vi "DOCK_save_database_password.vi"(7 "error_in":errorcluster, 9 "new_password":string, 10 "all_config_info_in":T1={"main_ini_file"={"SQL Driver"="", "SQL Server"="", "SQL Database"="", "SQL UID"="", "Reference table"="", "Reference history"="", "Archivisation CFG table"="", "Archivisation CFG history"="", "User table"="", "User history"="", "default language"="", "SCANNER COM port"=0, "SCANNER Baud rate"=0, "SCANNER Data bits"=0, "SCANNER Pairity"=enum."None", "SCANNER Stop bits"=0, "SCANNER Flow control"=0, "SCANNER Termination char"=10, "PRINTER PC port"=0, "PRINTER IP"="", "PRINTER port"=0, "PRINTER Keep alive timer [ms]"=0, "logout timeout [ms]"=0}, "SQL Password"="", "PRINTER Label"="", "PRINTER Template"="", "Last Label"="", "queue_refnums"={"MAIN_queue"=refnum, "SCANNER_queue"=refnum, "SCANNER_login"=refnum, "PRINTER_queue"=refnum}} {"main_ini_file"."SCANNER Flow control" items=["None"=0, "XON/XOFF"=1, "RTS/CTS"=2, "DTR/DSR"=4]; "main_ini_file"."SCANNER Stop bits" items=["1.0"=10, "1.5"=15, "2.0"=20]}) -> (0 "error_out":errorcluster, 3 "all_config_info_out":T1={"main_ini_file"={"SQL Driver"="", "SQL Server"="", "SQL Database"="", "SQL UID"="", "Reference table"="", "Reference history"="", "Archivisation CFG table"="", "Archivisation CFG history"="", "User table"="", "User history"="", "default language"="", "SCANNER COM port"=0, "SCANNER Baud rate"=0, "SCANNER Data bits"=0, "SCANNER Pairity"=enum."None", "SCANNER Stop bits"=0, "SCANNER Flow control"=0, "SCANNER Termination char"=10, "PRINTER PC port"=0, "PRINTER IP"="", "PRINTER port"=0, "PRINTER Keep alive timer [ms]"=0, "logout timeout [ms]"=0}, "SQL Password"="", "PRINTER Label"="", "PRINTER Template"="", "Last Label"="", "queue_refnums"={"MAIN_queue"=refnum, "SCANNER_queue"=refnum, "SCANNER_login"=refnum, "PRINTER_queue"=refnum}} {"main_ini_file"."SCANNER Flow control" items=["None"=0, "XON/XOFF"=1, "RTS/CTS"=2, "DTR/DSR"=4]; "main_ini_file"."SCANNER Stop bits" items=["1.0"=10, "1.5"=15, "2.0"=20]})   [LabVIEW 2019]
uses:
  ini/typedef/DOCK_all_config_info.ctl
  ini/typedef/DOCK_main_ini_file.ctl
  queues/typedef/DOCK_queue_refnums.ctl
  queues/typedef/DOCK_MAIN_queue_element.ctl
  MAIN/DOCK_MAIN_sequence_state.ctl
  queues/typedef/DOCK_SCANNER_queue_element.ctl
  SCANNER/DOCK_SCANNER_sequence_state.ctl
  queues/typedef/DOCK_PRINTER_queue_element.ctl
  PRINTER/DOCK_PRINTER_sequence_state.ctl
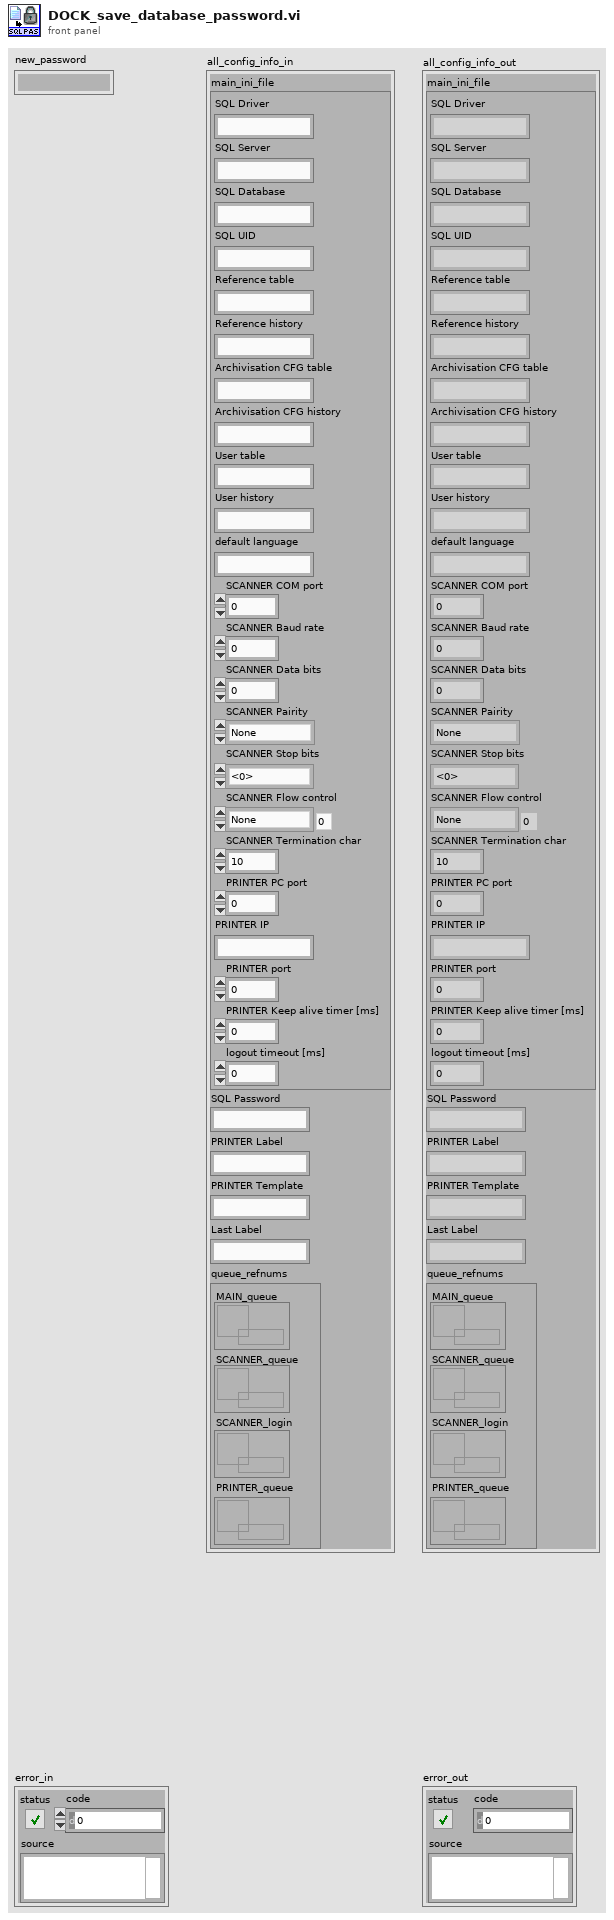
[diagram p1: front panel]
types:
  T1 = typedef "DOCK_all_config_info.ctl" = cluster{"main_ini_file":T2, "SQL Password":string, "PRINTER Label":string, "PRINTER Template":string, "Last Label":string, "queue_refnums":T3}
  T2 = typedef "DOCK_main_ini_file.ctl" = cluster{"SQL Driver":string, "SQL Server":string, "SQL Database":string, "SQL UID":string, "Reference table":string, "Reference history":string, "Archivisation CFG table":string, "Archivisation CFG history":string, "User table":string, "User history":string, "default language":string, "SCANNER COM port":u16, "SCANNER Baud rate":u32, "SCANNER Data bits":u16, "SCANNER Pairity":enum16{"None", "Odd", "Even", "Mark", "Space"}, "SCANNER Stop bits":u16, "SCANNER Flow control":u16, "SCANNER Termination char":u8, "PRINTER PC port":u16, "PRINTER IP":string, "PRINTER port":u16, "PRINTER Keep alive timer [ms]":i32, "logout timeout [ms]":i32}
  T3 = typedef "DOCK_queue_refnums.ctl" = cluster{"MAIN_queue":refnum<queue>, "SCANNER_queue":refnum<queue>, "SCANNER_login":refnum<queue>, "PRINTER_queue":refnum<queue>}
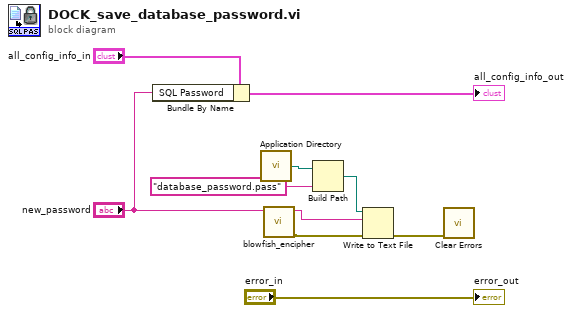
[diagram p0: block diagram]
diagram:
  n1 = Bundle By Name(cluster="all_config_info_in", "SQL Password"="new_password") -> (→"all_config_info_out":T1)
  n2 = call <vilib>:"Application Directory.vi"() -> ("Application Directory"=w9:path)
  n3 = call "blowfish_encipher.vi"("Input Text"="new_password") -> ("error out"=w5:errorcluster, "Output Text"=w4:string)  [unwired: 9 in]
  n4 = Build Path(base path=w9, name or relative path="database_password.pass") -> (appended path=w7:path)
  n5 = Write to Text File(file (use dialog)=w7, text=w4, error in=w5) -> (error out=w6:errorcluster)  [unwired: 1 in, 2 out]
  n6 = call <vilib>:"Clear Errors.vi"("error in (no error)"=w6) -> ()  [unwired: 5 in, 2 out]
  "error_out" <- "error_in"
